vi "Main.vi"() -> ()   [LabVIEW 2020]
panel:
  in  "stop":bool
  in  "Tab Control":T1(tab)
  out "XYグラフ":T2(graph)
  in  "Select Mol Posi":u16(ring)=4 items=["3 molecules", "5 molecules", "7 molecules", "9 molecules", "13 molecules", "17 molecules", ""]
  out "Particle State":T3(array[cluster])
  in  "SD":dbl=0.11000000000000001
  in  "Tau_On":i32=40
  in  "Tau_Off":i32=10
  in  "Sim_Time":i32=100000
  in  "Asymmetry (X, Y)":dbl[](array[numeric])=[0.12000000000000001, 0.58]
  out "Count":i32
  in  "Torque":bool=TRUE
  in  "Torque":dbl=-4.0
  out "Center State at T":T4
  in  "停止":bool
  in  "Rot_Noise for Cargo":bool
  in  "Width of Rot_Noise":dbl format="%#_13g"
  in  "Ini_Posi (3 mol)":dbl[][](array[numeric])=[[0.0, 0.0], [6.0, 0.0], [-6.0, 0.0]]
  in  "Ini_Posi (5 mol)":dbl[][](array[numeric])=[[0.0, 0.0], [6.0, 0.0], [-6.0, 0.0], [0.0, 6.0], [0.0, -6.0]]
  in  "Ini_Posi (9 mol)":dbl[][](array[numeric])=[[0.0, 0.0], [6.0, 0.0], [-6.0, 0.0], [0.0, 6.0], [0.0, -6.0], [6.0, 6.0], [6.0, -6.0], [-6.0, 6.0], [-6.0, -6.0]]
  in  "Ini_Posi (13 mol)":dbl[][](array[numeric])=[[0.0, 0.0], [6.0, 0.0], [-6.0, 0.0], [0.0, 6.0], [0.0, -6.0], [6.0, 6.0], [6.0, -6.0], [-6.0, 6.0], [-6.0, -6.0], [3.0, 3.0], [3.0, -3.0], [-3.0, 3.0], [-3.0, -3.0]]
  in  "Ini_Posi (13 mol#2)":dbl[][](array[numeric])=[[0.0, 0.0], [12.0, 3.0], [-12.0, 3.0], [12.0, -3.0], [-12.0, -3.0], [6.0, 0.0], [-6.0, 0.0], [0.0, -6.0], [0.0, 6.0], [6.0, 6.0], [6.0, -6.0], [-6.0, 6.0], [-6.0, -6.0], [3.0, 3.0], [3.0, -3.0], [-3.0, 3.0], [-3.0, -3.0]]
  in  "Ini_Posi (7 mol)":dbl[][](array[numeric])=[[0.0, 0.0], [5.0, 3.0], [-5.0, 3.0], [5.0, -3.0], [-5.0, -3.0], [0.0, 6.0], [0.0, -6.0]]
  out "Y":dbl[](graph)
  in  "# of filaments":dbl=13.0
  out "Trajectory":cluster{"Position":dbl[], "Position":dbl[]}[](graph)
  out "Angle":dbl[](graph)
  out "Expanded Trajectory":cluster{"Position":dbl[], "Position":dbl[]}[](graph)
  in  "OK Button":bool
  out "Num of On-Particles":dbl[](graph)
  out "Cross Corr":cluster{i32[], "Cross":dbl[]}(graph)
  out "Corr_Coef_Pearson":T5
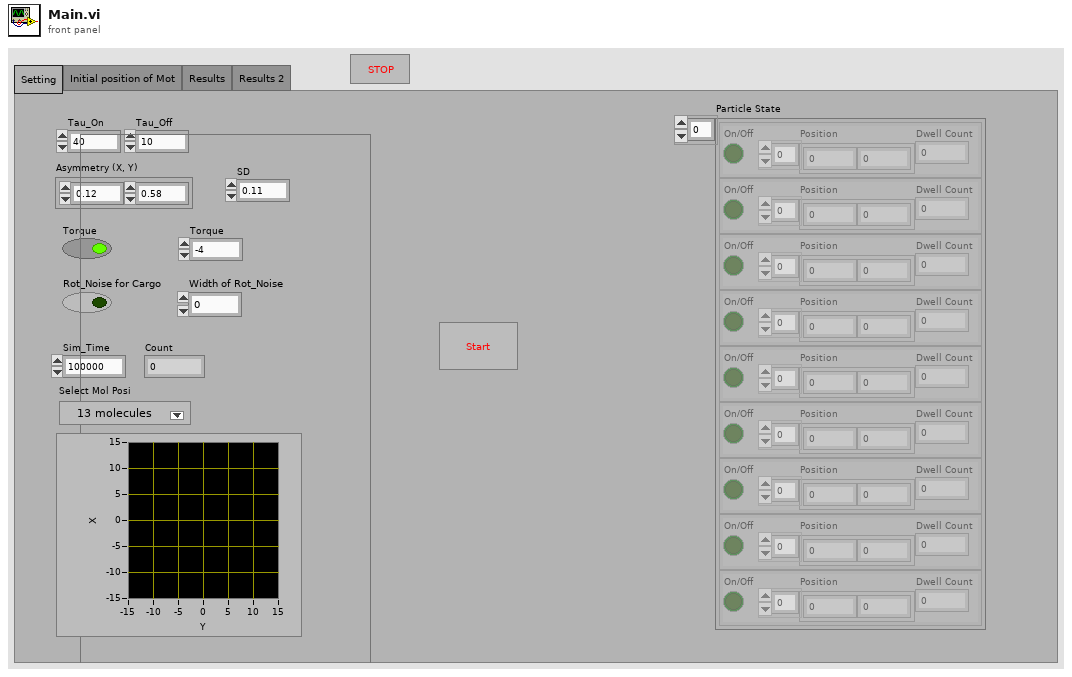
[diagram p1: front panel]
types:
  T1 = enum32{"Setting", "Initial position of Mot", "Results", "Results 2"}
  T2 = cluster{"Ini_Anchor_Posi (17 mol)":dbl[], "Ini_Anchor_Posi (17 mol)":dbl[]}
  T3 = cluster{"On/Off":bool, "Position":dbl[], "Dwell Count":i32}[]
  T4 = cluster{"Center Position":dbl[], "Center Angle":dbl}
  T5 = cluster{"correlation coefficient r":dbl, "r^2":dbl}
  T6 = cluster{"Ini_Posi (13 mol#2)":dbl[], "Ini_Posi (13 mol#2)":dbl[]}
  T7 = cluster{"On/Off":bool, "Position":dbl[], "Next Dwell":i32}[]
  T8 = cluster{"On/Off":bool, "Position":dbl[], "Next Dwell":i32}
  T9 = enum16{"open", "replace", "create", "open or create", "replace or create", "replace or create with confirmation"}
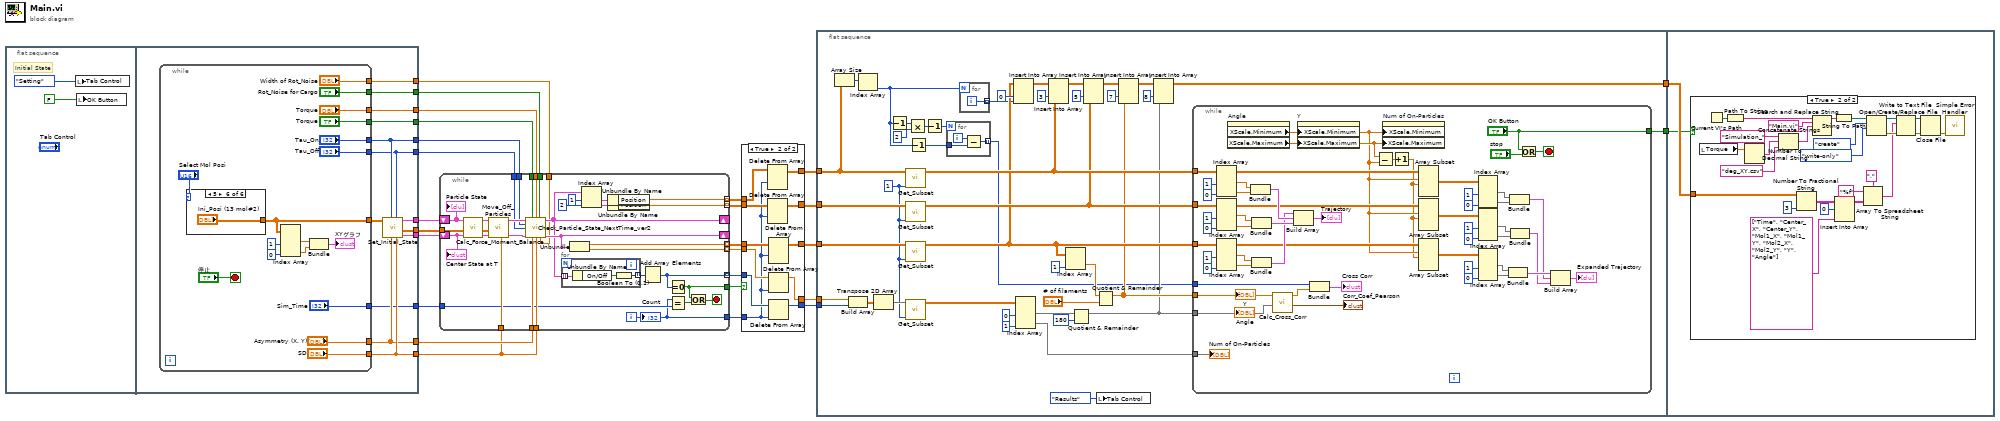
[diagram p0: block diagram]
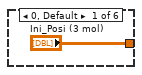
[diagram p4: hidden frame]
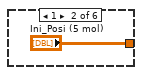
[diagram p5: hidden frame]
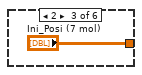
[diagram p6: hidden frame]
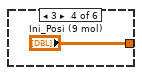
[diagram p7: hidden frame]
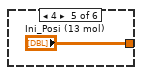
[diagram p8: hidden frame]
diagram:
  n1 = flat-sequence {
    tunnel: [w41] -> w26
    tunnel: [w40] -> w25
    tunnel: [w39] -> w24
    tunnel: [w36] -> w20
    tunnel: [w38] -> w23
    tunnel: [w37] -> w22
    tunnel: [w35] -> w21
    tunnel: [w34] -> w19
    tunnel: [w33] -> w18
    tunnel: [w31] -> w4
    tunnel: [w30] -> w3
    tunnel: [w29] -> w2
    frame #0 {
      # "Initial State"
      n2 = local write "Tab Control"(T1."Setting" ("Tab Control")) -> ()
      n3 = local write "OK Button"(FALSE ("OK Button")) -> ()
    }
    frame #1 {
      n4 = while {
        tunnel: ["Tau_On"] -> w38
        tunnel: ["Tau_Off"] -> w37
        tunnel: ["SD"] -> w36
        tunnel: ["Asymmetry (X, Y)"] -> w35
        tunnel: ["Torque"] -> w34
        tunnel: ["Torque"] -> w33
        tunnel: [w52] -> w32
        tunnel: ["Rot_Noise for Cargo"] -> w31
        tunnel: ["Width of Rot_Noise"] -> w30
        tunnel: ["Sim_Time"] -> w29
        stop <- "停止" stop-if-true
        n5 = case shown="5" "Select Mol Posi" {
          tunnel: ["Ini_Posi (3 mol)" "Ini_Posi (5 mol)" "Ini_Posi (7 mol)" "Ini_Posi (9 mol)" "Ini_Posi (13 mol)" "Ini_Posi (13 mol#2)"] -> w52
          frame 0, Default {
          }
          frame 1 {
          }
          frame 2 {
          }
          frame 3 {
          }
          frame 4 {
          }
          frame 5 {
          }
        }
        n6 = Index Array(array=w52, index (col) #1=1 ("無効な指標 (列)"), index (col) #2=0 ("指標 (列)")) -> (element #1=w47:dbl[], element #2=w46:dbl[])  [unwired: 2 in]
        n7 = Bundle("Ini_Posi (13 mol#2)"=w47, "Ini_Posi (13 mol#2)"=w46) -> (→"XYグラフ":T6)  [unwired: 1 in]
      }
      n8 = call "Set_Initial_State.vi"("SD"=w36, "Tau_Off"=w37, "Asymmetry (X, Y)"=w35, "Tau_On"=w38, "Ini_Anchor_Posi"=w32) -> ("Center State at T"=w39:T4, "Ini_Anchor_Posi"=w40:dbl[][], "On_Particle State"=w41:T3)  [unwired: 4 in]
    }
  }
  n9 = while {
    tunnel: w25 -> [w97]
    shift-right: [w84] -> _
    shift-left: w24 -> [w95]
    shift-right: [w76] -> _
    shift-left: w26 -> [w96]
    tunnel: w20 -> [w89]
    tunnel: w23 -> [w83]
    tunnel: w22 -> [w82]
    tunnel: w21 -> [w79]
    tunnel: [w92] -> w14 mode=indexing
    tunnel: [w91] -> w13 mode=indexing
    tunnel: [w90] -> w12 mode=indexing
    tunnel: w20 -> [w78]
    tunnel: w19 -> [w80]
    tunnel: w18 -> [w81]
    tunnel: [w77] -> w11 mode=indexing
    tunnel: [w71] -> w10 mode=indexing
    tunnel: w2 -> [w72]
    tunnel: [w68] -> w15
    tunnel: [w67] -> w1
    tunnel: w4 -> [w66]
    tunnel: w3 -> [w65]
    i -> [w67]
    stop <- w69 stop-if-true
    n10 = call "Calc_Force_Moment_Balance.vi"("Center State at T"=w95, "Ini_Anchor_Posi"=w97, "On_Particle State"=w96) -> ("New Center State at T"=w86:T4, "Ini_Anchor_Posi"=w87:dbl[][], "On_Particle State"=w98:T3)  [unwired: 6 in]
    n11 = call "Move_Off_Particles.vi"("SD"=w89, "Center State at T"=w86, "Ini_Anchor_Posi"=w87, "Particle Posi at T"=w98) -> ("Center State at T"=w85:T4, "New Particle Posi at T"=w88:T7)  [unwired: 6 in]
    n12 = call "Check_Particle_State_NextTime_ver2.vi"("Particle State at T"=w88, "Torque?"=w80, "Torque"=w81, "Rot diffusion\nfor Cargo?"=w66, "Tau_On"=w83, "Tau_Off"=w82, "Center State at T"=w85, "Asymmetry (X, Y)"=w79, "SD"=w78, "Rot diffusion\nfor Cargo"=w65) -> ("Particle State at T+1"=w76:T7, "New Center State at T"=w84:T4)  [unwired: 4 in]
    n13 = for {
      tunnel: w76 -> [w101] mode=indexing
      tunnel: [w99] -> w75 mode=indexing
      n14 = Unbundle By Name(w101) -> ("On/Off"=w100:bool)
      n15 = Boolean To (0,1)(Boolean=w100) -> (0, 1=w99:i16)
    }
    n16 = Unbundle(w84) -> ("Center Position"=w90:dbl[], "Center Angle"=w77:dbl)
    n17 = Index Array(array=w76, index #1=1 ("index"), index #2=2 ("index")) -> (element #1=w94:T8, element #2=w93:T8)
    n18 = Unbundle By Name(w94) -> ("Position"=w92:dbl[])
    n19 = Unbundle By Name(w93) -> ("Position"=w91:dbl[])
    n20 = Add Array Elements(numeric array=w75) -> (sum=w71:i16)
    n21 = Equal To 0?(x=w71) -> (x = 0?=w68:bool)
    n22 = Equal?(x=w67, y=w72) -> (x = y?=w70:bool)
    n23 = Or(x=w68, y=w70) -> (x .or. y?=w69:bool)
    "Particle State" <- w96
    "Center State at T" <- w95
    "Count" <- w67
  }
  n24 = case shown="TRUE" w15 {
    tunnel: w14 -> [w106 w117]
    tunnel: w13 -> [w105 w116]
    tunnel: w1 -> [_ w112]
    tunnel: w12 -> [w104 w115]
    tunnel: w11 -> [w103 w114]
    tunnel: w10 -> [w102 w113]
    tunnel: [w102 w111] -> w9
    tunnel: [w103 w110] -> w8
    tunnel: [w104 w109] -> w7
    tunnel: [w105 w108] -> w6
    tunnel: [w106 w107] -> w5
    frame False {
    }
    frame True {
      n25 = Delete From Array(array=w117, index (row)=w112) -> (array with subset deleted=w107:dbl[][])  [unwired: 2 in, 1 out]
      n26 = Delete From Array(array=w116, index (row)=w112) -> (array with subset deleted=w108:dbl[][])  [unwired: 2 in, 1 out]
      n27 = Delete From Array(array=w115, index (row)=w112) -> (array with subset deleted=w109:dbl[][])  [unwired: 2 in, 1 out]
      n28 = Delete From Array(array=w114, index=w112) -> (array with subset deleted=w110:dbl[])  [unwired: 1 in, 1 out]
      n29 = Delete From Array(array=w113, index=w112) -> (array with subset deleted=w111:i16[])  [unwired: 1 in, 1 out]
    }
  }
  n30 = flat-sequence {
    tunnel: w5 -> [w127]
    tunnel: w6 -> [w160]
    tunnel: w7 -> [w159]
    tunnel: w8 -> [w158]
    tunnel: w9 -> [w152]
    tunnel: [w132] -> w17
    tunnel: [w149] -> w16
    tunnel: w17 -> [w218]
    tunnel: w16 -> [w217]
    frame #0 {
      w128 = 1
      n31 = Array Size(array=w127) -> (size(s)=w126:i32[])
      n32 = Build Array(w158, w152) -> (w157:dbl[][])
      n33 = Index Array(array=w126) -> (element=w121:i32)  [unwired: 1 in]
      n34 = Transpose 2D Array(2D array=w157) -> (transposed array=w156:dbl[][])
      n35 = Decrement(x=w121) -> (x-1=w120:i32)
      n36 = call "Get_Subset.vi"("index"=w128, "Input"=w127) -> ("Output"=w147:dbl[][])  [unwired: 9 in]
      n37 = call "Get_Subset.vi"("index"=w128, "Input"=w160) -> ("Output"=w144:dbl[][])  [unwired: 9 in]
      n38 = call "Get_Subset.vi"("index"=w128, "Input"=w159) -> ("Output"=w140:dbl[][])  [unwired: 9 in]
      n39 = call "Get_Subset.vi"("index"=w128, "Input"=w156) -> ("Output"=w155:dbl[][])  [unwired: 9 in]
      n40 = Multiply(x=w120, y=2) -> (x*y=w122:i32)
      n41 = Decrement(x=w121) -> (x-1=w118:i32)
      n42 = Decrement(x=w122) -> (x-1=w119:i32)
      n43 = for {
        N: w119 -> [_]
        tunnel: [w162] -> w123 mode=indexing
        tunnel: w118 -> [w161]
        i -> [w163]
        n44 = Subtract(x=w163, y=w161) -> (x-y=w162:i32)
      }
      n45 = for {
        N: w121 -> [_]
        tunnel: [w164] -> w125 mode=indexing
        i -> [w164]
      }
      n46 = Insert Into Array(array=w140, index (col)=0 ("disabled index (col)"), new element=w125) -> (w148:dbl[][])  [unwired: 1 in]
      n47 = Index Array(array=w155, index (col) #1=0 ("disabled index (col)"), index (col) #2=1 ("index (col)")) -> (element #1=w141:dbl[], element #2=w151:dbl[])  [unwired: 2 in]
      n48 = Insert Into Array(array=w148, index (col)=3 ("disabled index (col)"), new element=w147) -> (w145:dbl[][])  [unwired: 1 in]
      n49 = Index Array(array=w140, index (col)=1 ("disabled index (col)")) -> (element=w138:dbl[])  [unwired: 1 in]
      n50 = Quotient & Remainder(x=w141, y=180) -> (x-y*floor(x/y)=w131:dbl[])  [unwired: 1 out]
      n51 = Insert Into Array(array=w145, index (col)=5 ("disabled index (col)"), new element=w144) -> (w136:dbl[][])  [unwired: 1 in]
      n52 = Quotient & Remainder(x=w138, y="# of filaments") -> (x-y*floor(x/y)=w135:dbl[])  [unwired: 1 out]
      n53 = local write "Tab Control"(T1."Results" ("Tab Control")) -> ()
      n54 = Insert Into Array(array=w136, index (col)=7 ("disabled index (col)"), new element=w135) -> (w133:dbl[][])  [unwired: 1 in]
      n55 = Insert Into Array(array=w133, index (col)=8 ("disabled index (col)"), new element=w131) -> (w132:dbl[][])  [unwired: 1 in]
      n56 = while {
        tunnel: w147 -> [w201]
        tunnel: w144 -> [w198]
        tunnel: w140 -> [w197]
        tunnel: w151 -> [w202]
        tunnel: ["OK Button"] -> w149
        tunnel: w131 -> [w169]
        tunnel: w135 -> [w170]
        tunnel: w123 -> [w166]
        stop <- w173 stop-if-true
        n57 = Index Array(array=w201, index (col) #1=1 ("disabled index (col)"), index (col) #2=0 ("index (col)")) -> (element #1=w203:dbl[], element #2=w212:dbl[])  [unwired: 2 in]
        n58 = Index Array(array=w198, index (col) #1=1 ("disabled index (col)"), index (col) #2=0 ("index (col)")) -> (element #1=w204:dbl[], element #2=w211:dbl[])  [unwired: 2 in]
        n59 = Index Array(array=w197, index (col) #1=1 ("disabled index (col)"), index (col) #2=0 ("index (col)")) -> (element #1=w171:dbl[], element #2=w206:dbl[])  [unwired: 2 in]
        n60 = property on="Angle" class="WFGraph (指定)"() -> ("XScale.Minimum"=w176:dbl, "XScale.Maximum"=w200:dbl)  [unwired: 2 in, 2 out]
        n61 = Bundle("Output"=w203, "Output"=w212) -> (w210:cluster{"Output":dbl[], "Output":dbl[]})  [unwired: 1 in]
        n62 = Bundle("Output"=w204, "Output"=w211) -> (w209:cluster{"Output":dbl[], "Output":dbl[]})  [unwired: 1 in]
        n63 = Bundle("Output"=w171, "Output"=w206) -> (w205:cluster{"Output":dbl[], "Output":dbl[]})  [unwired: 1 in]
        n64 = call "Calc_Cross_Corr.vi"("Y"=w169, "X"=w170) -> ("Corr_Coef_Pearson"=→"Corr_Coef_Pearson":T5, "Cross"=w167:dbl[])  [unwired: 7 in, 1 out]
        n65 = Build Array(w205, w210, w209) -> (→"Trajectory":cluster{"Output":dbl[], "Output":dbl[]}[])
        n66 = property on="Y" class="WFGraph (指定)"("XScale.Minimum"=w176, "XScale.Maximum"=w200) -> ()  [unwired: 2 in, 2 out]
        n67 = Bundle(w166, "Cross"=w167) -> (→"Cross Corr":cluster{i32[], "Cross":dbl[]})  [unwired: 1 in]
        n68 = Subtract(x=w200, y=w176) -> (x-y=w199:dbl)
        n69 = property on="Num of On-Particles" class="WFGraph (指定)"("XScale.Minimum"=w176, "XScale.Maximum"=w200) -> ()  [unwired: 2 in, 2 out]
        n70 = Increment(x=w199) -> (x+1=w175:dbl)
        n71 = Array Subset(array=w201, index (row)=w176, length (row)=w175) -> (w178:dbl[][])  [unwired: 2 in]
        n72 = Array Subset(array=w198, index (row)=w176, length (row)=w175) -> (w177:dbl[][])  [unwired: 2 in]
        n73 = Array Subset(array=w197, index (row)=w176, length (row)=w175) -> (w179:dbl[][])  [unwired: 2 in]
        n74 = Index Array(array=w178, index (col) #1=1 ("disabled index (col)"), index (col) #2=0 ("index (col)")) -> (element #1=w190:dbl[], element #2=w189:dbl[])  [unwired: 2 in]
        n75 = Index Array(array=w177, index (col) #1=1 ("disabled index (col)"), index (col) #2=0 ("index (col)")) -> (element #1=w188:dbl[], element #2=w187:dbl[])  [unwired: 2 in]
        n76 = Index Array(array=w179, index (col) #1=1 ("disabled index (col)"), index (col) #2=0 ("index (col)")) -> (element #1=w186:dbl[], element #2=w185:dbl[])  [unwired: 2 in]
        n77 = Bundle(w186, w185) -> (w184:cluster{dbl[], dbl[]})  [unwired: 1 in]
        n78 = Bundle(w190, w189) -> (w183:cluster{dbl[], dbl[]})  [unwired: 1 in]
        n79 = Bundle(w188, w187) -> (w182:cluster{dbl[], dbl[]})  [unwired: 1 in]
        n80 = Or(x="OK Button", y="stop") -> (x .or. y?=w173:bool)
        n81 = Build Array(w184, w183, w182) -> (→"Expanded Trajectory":cluster{dbl[], dbl[]}[])
        "Angle" <- w169
        "Y" <- w170
        "Num of On-Particles" <- w202
      }
    }
    frame #1 {
      n82 = case shown="TRUE" w217 {
        tunnel: w218 -> [_ w228]
        frame False {
        }
        frame True {
          n83 = local read "Torque"() -> (w227:dbl)
          n84 = Current VI's Path() -> (path=w223:path)
          n85 = Path To String(path=w223) -> (string=w222:string)
          n86 = Number To Decimal String(number=w227) -> (decimal integer string=w225:string)  [unwired: 1 in]
          n87 = Concatenate Strings("Simulation_" ("文字列"), w225, "deg_XY.csv" ("string")) -> (w220:string)
          n88 = Number To Fractional String(number=w228, precision (6)=i16 3) -> (F-format string=w236:string[][])  [unwired: 2 in]
          n89 = Search and Replace String(input string=w222, search string="Main.vi", replace string=w220) -> (result string=w219:string)  [unwired: 5 in, 3 out]
          n90 = String To Path(string=w219) -> (path=w237:path)
          n91 = Insert Into Array(array=w236, index (row)=0, new element=string[] ["Time", "Center_X", "Center_Y", "Mol1_X", "Mol1_Y", "Mol2_X", "Mol2_Y", "Y", "Angle"]) -> (w234:string[][])  [unwired: 1 in]
          n92 = Array To Spreadsheet String(delimiter (Tab)=",", array=w234, 3:"%f" ("format string")) -> (spreadsheet string=w232:string)
          n93 = Open/Create/Replace File(file path (use dialog)=w237, operation (0:open)=T9."create", access (0:read/write)=enum16{"read/write", "read-only", "write-only"}."write-only") -> (refnum out=w240:refnum<file>, error out=w241:errorcluster)  [unwired: 1 in, 3 out]
          n94 = Write to Text File(file (use dialog)=w240, text=w232, error in=w241) -> (refnum out=w243:refnum<file>, error out=w244:errorcluster)  [unwired: 1 in, 1 out]
          n95 = Close File(refnum=w243, error in=w244) -> (error out=w242:errorcluster)  [unwired: 1 out]
          n96 = call <vilib>:"Simple Error Handler.vi"("error in (no error)"=w242) -> ()  [unwired: 1 in, 8 out]
        }
      }
    }
  }
